vi "NewCore.vi"(8 "error in (no error)":errorcluster, 11 "MazeGame":refnum<class "MazeGame.lvclass">) -> (0 "error out":errorcluster, 3 "MazeGame":refnum<class "MazeGame.lvclass">)   [LabVIEW 2020, in "FactoryMethod.lvlib" / "MazeGame.lvclass"]
uses:
  MazeGame.lvclass
  Private/TypeDef/privateData.ctl
  MazeGame.lvclass/MazeGame.ctl
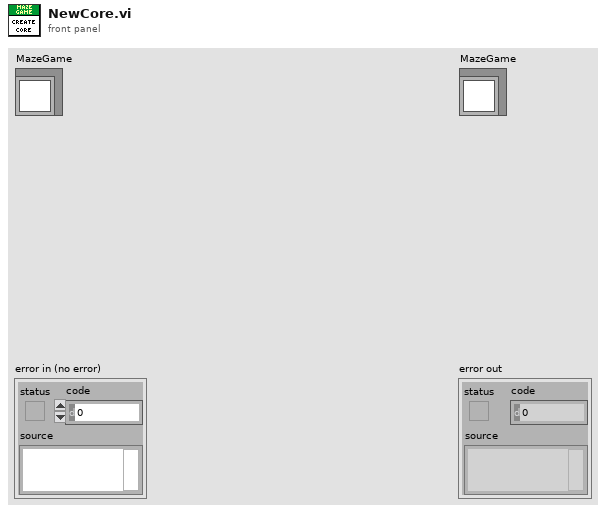
[diagram p1: front panel]
types:
  T1 = typedef "FactoryMethod.lvlib/MazeGame.lvclass/privateData.ctl" = cluster{"Dummy":i32}
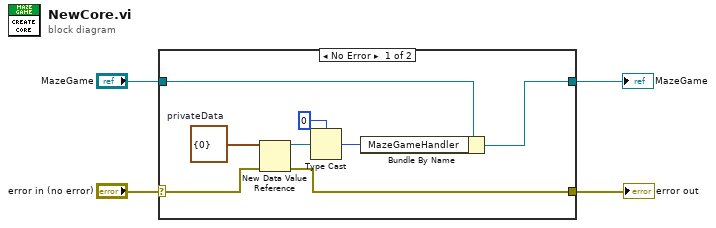
[diagram p0: block diagram]
diagram:
  n1 = case shown="No Error" "error in (no error)" {
    selector: "error in (no error)" -> [w6 w14]
    tunnel: [w7 w14] -> w3
    tunnel: [w9 w13] -> w4
    tunnel: "MazeGame" -> [w8 w13]
    frame No Error {
      w5 = T1 {"Dummy"=0}  # privateData
      n2 = New Data Value Reference(data value=w5, error in=w6) -> (data value reference=w12:refnum<data-value>, error out=w7:errorcluster)
      n3 = Type Cast(type=u32 0, x=w12) -> (*(type *) &x=w10:u32)
      n4 = Bundle By Name(cluster=w8, "MazeGameHandler"=w10) -> (w9:refnum<class "MazeGame.lvclass">)
    }
    frame Error {
    }
  }
  "error out" <- w3
  "MazeGame" <- w4
